vi "CMD_Drive.vi"(1 "Line":string) -> (0 "Done":bool)   [LabVIEW 2013]
uses:
  <vilib>/addons/control/pid/pid.llb/PID (DBL).vi
  <vilib>/addons/control/pid/NI_PID_pid.lvlib
panel:
  in  "Parameters":i32[](array[numeric])=[1, 3, 1, 3, 1]
  in  "Subcommands":string[](array[string])=["at", "at", "for", "to", "until"]
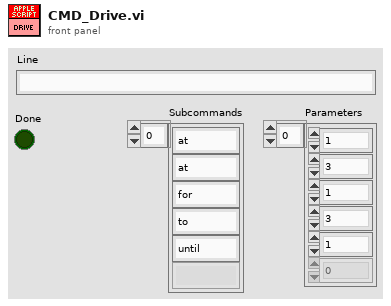
[diagram p1: front panel]
types:
  T1 = cluster{"proportional gain (Kc)":dbl, "integral time (Ti, min)":dbl, "derivative time (Td, min)":dbl}
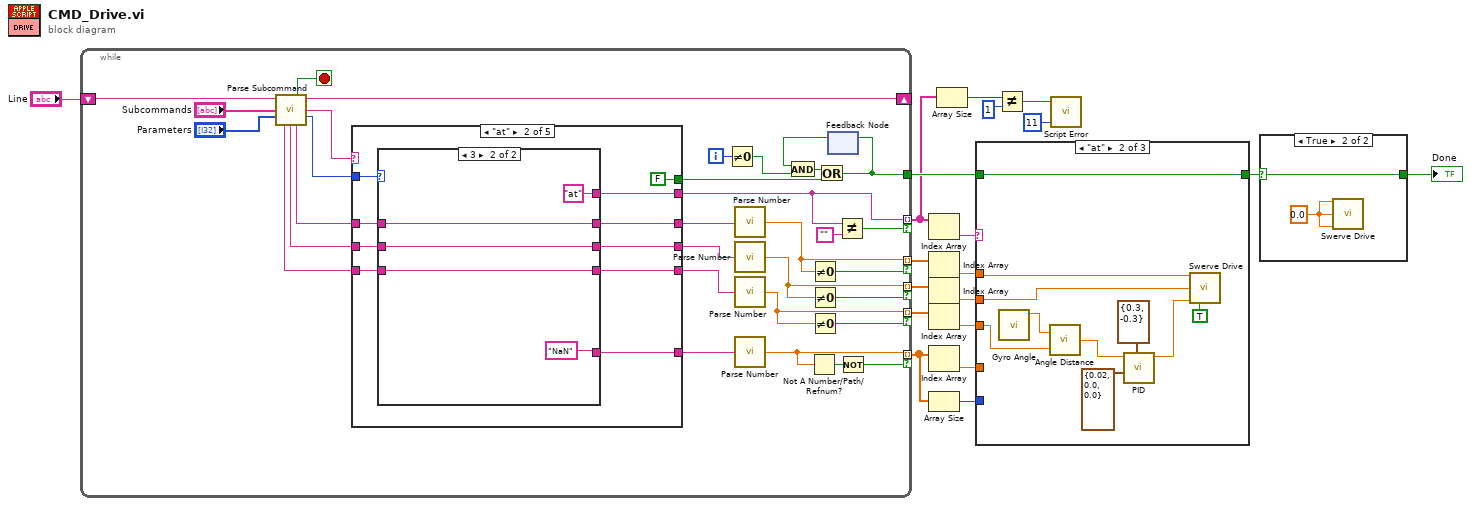
[diagram p0: block diagram]
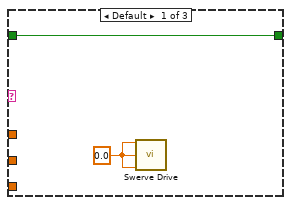
[diagram p3: hidden frame]
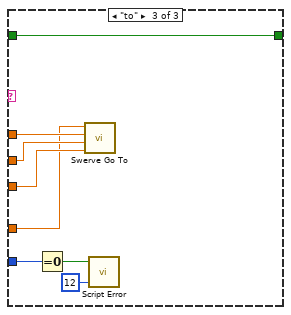
[diagram p4: hidden frame]
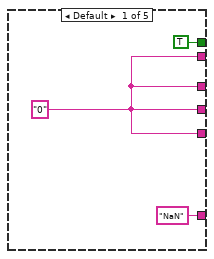
[diagram p5: hidden frame]
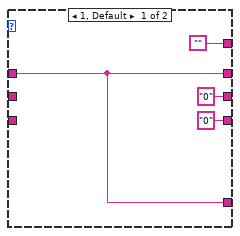
[diagram p6: hidden frame]
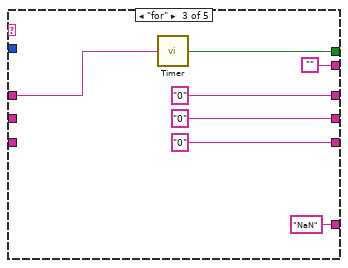
[diagram p7: hidden frame]
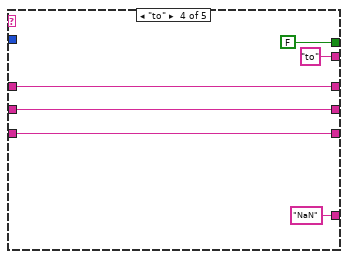
[diagram p8: hidden frame]
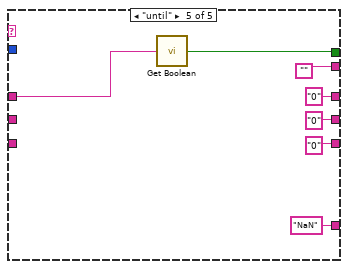
[diagram p9: hidden frame]
diagram:
  n1 = while {
    shift-right: [w48] -> _
    shift-left: "Line" -> [w51]
    tunnel: [w39] -> w4
    tunnel: [w31] -> w16 mode=indexing if=w25
    tunnel: [w30] -> w14 mode=indexing if=w23
    tunnel: [w27] -> w12 mode=indexing if=w24
    tunnel: [w22] -> w2 mode=indexing if=w20
    tunnel: [w33] -> w3 mode=indexing if=w34
    i -> [w36]
    stop <- w47 stop-if-true
    n2 = call "Parse Subcommand.vi"("Text In"=w51, "Subcommands"="Subcommands", "Parameters"="Parameters") -> ("Done"=w47:bool, "Text Out"=w48:string, "Subcommand"=w46:string, "# of Parameters"=w45:i32, "Parameter 3"=w43:string, "Parameter 2"=w42:string, "Parameter 1"=w44:string)  [unwired: 6 in]
    n3 = case shown="\"at\"" w46 {
      tunnel: w45 -> [_ w64 _ _ _]
      tunnel: w44 -> [_ w63 w74 w86 w88]
      tunnel: w42 -> [_ w62 _ w85 _]
      tunnel: w43 -> [_ w61 _ w84 _]
      tunnel: [w53 w60 "0" ("Parameter 1") w86 "0" ("Parameter 1")] -> w32
      tunnel: [w53 w59 "0" ("Parameter 2") w85 "0" ("Parameter 1")] -> w29
      tunnel: [w53 w58 "0" ("Parameter 3") w84 "0" ("Parameter 1")] -> w28
      tunnel: [TRUE ("Value") FALSE ("Running") w75 FALSE w87] -> w40
      tunnel: [w53 w55 "" "to" ("format string") ""] -> w33
      tunnel: ["NaN" ("Parameter 1") w57 "NaN" ("Parameter 3") "NaN" ("Parameter 3") "NaN" ("Parameter 1")] -> w26
      frame Default {
        w53 = "0" ("format string")
      }
      frame "at" {
        n4 = case shown="3" w64 {
          tunnel: w63 -> [w66 w73]
          tunnel: w62 -> [_ w72]
          tunnel: w61 -> [_ w69]
          tunnel: [w66 w73] -> w60
          tunnel: ["0" ("Parameter 2") w72] -> w59
          tunnel: ["0" ("Parameter 3") w69] -> w58
          tunnel: [w66 "NaN" ("Parameter 3")] -> w57
          tunnel: ["" "at"] -> w55
          frame 1, Default {
          }
          frame 3 {
          }
        }
      }
      frame "for" {
        n5 = call "Timer.vi"("Seconds (string)"=w74) -> ("Done"=w75:bool)
      }
      frame "to" {
      }
      frame "until" {
        n6 = call "Get Boolean.vi"("Name"=w88) -> ("Value"=w87:bool)
      }
    }
    n7 = Not Equal To 0?(x=w36) -> (x != 0?=w35:bool)
    n8 = call "Parse Number.vi"("String"=w32) -> ("Number"=w31:dbl)
    n9 = call "Parse Number.vi"("String"=w29) -> ("Number"=w30:dbl)
    n10 = call "Parse Number.vi"("String"=w28) -> ("Number"=w27:dbl)
    n11 = call "Parse Number.vi"("String"=w26) -> ("Number"=w22:dbl)
    n12 = Not A Number/Path/Refnum?(number/path/refnum=w22) -> (NaN/Path/Refnum?=w21:bool)
    n13 = Not Equal To 0?(x=w31) -> (x != 0?=w25:bool)
    n14 = Not Equal To 0?(x=w30) -> (x != 0?=w23:bool)
    n15 = Not Equal To 0?(x=w27) -> (x != 0?=w24:bool)
    n16 = feedback #1() -> (w37:bool)  [unwired: 1 in]
    n17 = And(x=w37, y=w35) -> (x .and. y?=w38:bool)
    n18 = Or(x=w38, y=w40) -> (x .or. y?=w39:bool)
    n19 = feedback-in #1(w39) -> ()
    n20 = Not Equal?(x=w33, y="") -> (x != y?=w34:bool)
    n21 = Not(x=w21) -> (.not. x?=w20:bool)
  }
  n22 = Index Array(array=w3) -> (element=w9:string)  [unwired: 1 in]
  n23 = Index Array(array=w16) -> (element=w15:dbl)  [unwired: 1 in]
  n24 = Index Array(array=w14) -> (element=w13:dbl)  [unwired: 1 in]
  n25 = Index Array(array=w12) -> (element=w11:dbl)  [unwired: 1 in]
  n26 = Index Array(array=w2) -> (element=w10:dbl)  [unwired: 1 in]
  n27 = Array Size(array=w2) -> (size(s)=w1:i32)
  n28 = Array Size(array=w3) -> (size(s)=w7:i32)
  n29 = case shown="\"at\"" w9 {
    tunnel: w15 -> [_ w96 w112]
    tunnel: w4 -> [w95 w105 w113]
    tunnel: [w95 w105 w113] -> w17
    tunnel: w13 -> [_ w104 w111]
    tunnel: w11 -> [_ w99 w110]
    tunnel: w10 -> [_ _ w109]
    tunnel: w1 -> [_ _ w107]
    frame Default {
      w94 = 0.0 ("X")
      n30 = call "Swerve Drive.vi"("X"=w94, "Y"=w94, "Z"=w94) -> ()  [unwired: 13 in]
    }
    frame "at" {
      n31 = call "Gyro Angle.vi"() -> ("Angle"=w100:dbl)  [unwired: 10 in, 1 out]
      n32 = call "Angle Distance.vi"("target angle"=w99, "current angle"=w100) -> ("distance"=w98:dbl)
      n33 = call-poly <vilib>:"PID.vi"("output range"=cluster{"output high":dbl, "output low":dbl} {"output high"=0.3, "output low"=-0.3}, "PID gains"=T1 {"proportional gain (Kc)"=0.02, "integral time (Ti, min)"=0.0, "derivative time (Td, min)"=0.0}, "setpoint"=w98) -> ("output"=w97:dbl)  [unwired: 7 in, 1 out]
      n34 = call "Swerve Drive.vi"("X"=w96, "Y"=w104, "Z"=w97, "Auto Controls"=TRUE) -> ()  [unwired: 12 in]
    }
    frame "to" {
      n35 = Equal To 0?(x=w107) -> (x = 0?=w106:bool)
      n36 = call "Swerve Go To.vi"("Max Speed"=w109, "Target X"=w112, "Target Y"=w111, "Target Angle"=w110) -> ()  [unwired: 3 in, 1 out]
      n37 = call "Script Error.vi"("Error?"=w106, "Error Code"=12) -> ()  [unwired: 4 in]
    }
  }
  n38 = Not Equal?(x=w7, y=1) -> (x != y?=w5:bool)
  n39 = call "Script Error.vi"("Error?"=w5, "Error Code"=11) -> ()  [unwired: 4 in]
  n40 = case shown="True" w17 {
    selector: w17 -> [w114 w116]
    tunnel: [w114 w116] -> w18
    frame False {
    }
    frame True {
      w115 = 0.0 ("X")
      n41 = call "Swerve Drive.vi"("X"=w115, "Y"=w115, "Z"=w115) -> ()  [unwired: 13 in]
    }
  }
  "Done" <- w18
